vi "Execute Eulogy.vi"(6 "Mouse Position":T1, 8 "User VI Ref":refnum<vi>, 9 "Menu Item Tag Suffix":string, 10 "Remaining Items":refnum<vi>[](array[refnum]), 11 "Affected Items":T2) -> (0 "Fail transaction?":bool)   [LabVIEW 2018, in "Shortcut Menu.lvlib"]
doc: "This VI is part of a plug-in for modifying the LabVIEW shortcut menus. This is the execute VI which is called when the shortcut menu is chosen by the user. It performs the action of the selected menu item."
uses:
  Shortcut Menu.lvlib
  Eulogy.ctl
  <vilib>/Utility/miscctls.llb/LVPositionTypeDef.ctl
  Toolkit/Toolkit.lvlib
panel:
  # "All controls on this panel except \"Affected Items\" have been locked to prevent accidental edits. Changing the control names or types, other than the elements of the \"Affected Items\" cluster will make the VI unusable as a menu plugin.\n\nSee Context Help for each control for details about its use."
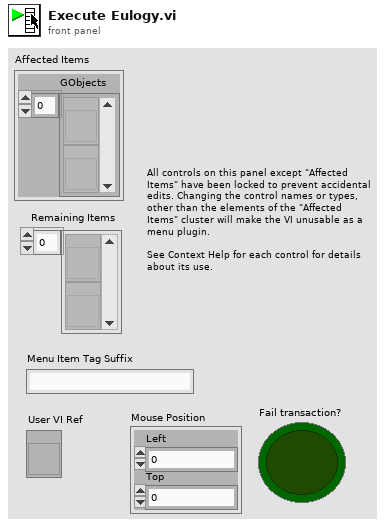
[diagram p1: front panel]
types:
  T1 = typedef "LVPositionTypeDef.ctl" = cluster{"Left":i32, "Top":i32}
  T2 = typedef "Shortcut Menu.lvlib/Eulogy.ctl" = cluster{"GObjects":refnum<vi>[]}
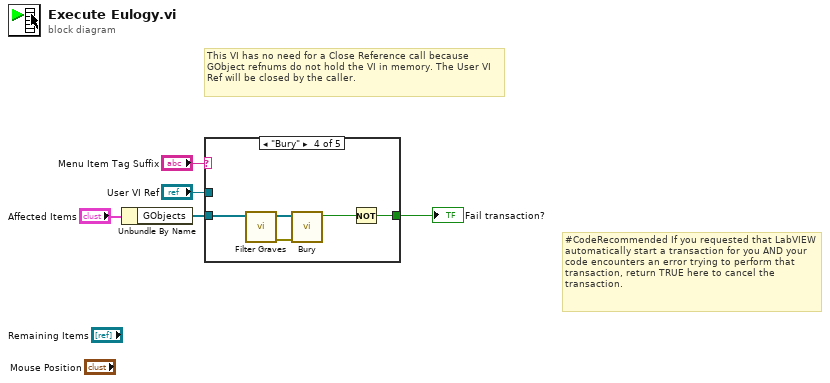
[diagram p0: block diagram]
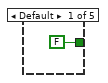
[diagram p2: hidden frame]
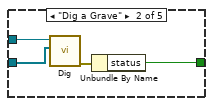
[diagram p3: hidden frame]
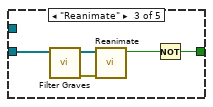
[diagram p4: hidden frame]
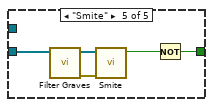
[diagram p5: hidden frame]
diagram:
  # "#CodeRecommended If you requested that LabVIEW automatically start a transaction for you AND your code encounters an error trying to perform that transaction, return TRUE here to cancel the transaction."
  # "This VI has no need for a Close Reference call because GObject refnums do not hold the VI in memory. The User VI Ref will be closed by the caller."
  n1 = Unbundle By Name("Affected Items") -> ("GObjects"=w2:refnum<vi>[])
  n2 = case shown="\"Bury\"" "Menu Item Tag Suffix" {
    tunnel: [FALSE ("Fail transaction?") w7 w11 w16 w21] -> w3
    tunnel: w2 -> [_ w10 w14 w20 w25]
    tunnel: "User VI Ref" -> [_ w9 _ _ _]
    frame Default {
    }
    frame "Dig a Grave" {
      n3 = call "Dig.vi"("Selection List[]"=w10, "VI In"=w9) -> ("Error Out"=w8:errorcluster)  [unwired: 8 in, 1 out]
      n4 = Unbundle By Name(w8) -> ("status"=w7:bool)
    }
    frame "Reanimate" {
      n5 = call "Filter Graves.vi"("GObjects"=w14) -> ("Error Out"=w12:errorcluster, "Graves"=w13:refnum<vi>[])  [unwired: 9 in]
      n6 = call "Reanimate.vi"("Error In"=w12, "Graves"=w13) -> ("Change Made?"=w15:bool)  [unwired: 8 in, 1 out]
      n7 = Not(x=w15) -> (.not. x?=w11:bool)
    }
    frame "Bury" {
      n8 = call "Filter Graves.vi"("GObjects"=w20) -> ("Error Out"=w18:errorcluster, "Graves"=w19:refnum<vi>[])  [unwired: 9 in]
      n9 = call "Bury.vi"("Error In"=w18, "Graves"=w19) -> ("Change Made?"=w17:bool)  [unwired: 8 in, 1 out]
      n10 = Not(x=w17) -> (.not. x?=w16:bool)
    }
    frame "Smite" {
      n11 = call "Filter Graves.vi"("GObjects"=w25) -> ("Error Out"=w23:errorcluster, "Graves"=w24:refnum<vi>[])  [unwired: 9 in]
      n12 = call "Smite.vi"("Error In"=w23, "Graves"=w24) -> ("Change Made?"=w22:bool)  [unwired: 8 in, 1 out]
      n13 = Not(x=w22) -> (.not. x?=w21:bool)
    }
  }
  "Fail transaction?" <- w3
